vi "Query Bandwidth Part.vi"(6 "Carrier Component (1)":T2=1, 8 "error in (no error)":errorcluster, 9 "Bandwidth Part (BWP0)":T1 items=["BWP0"], 10 "Instance (1)":T3=1, 11 "VISA resource name":refnum<visa-resource-name>) -> (0 "error out":errorcluster, 1 "Cyclic Prefix":i32(ring) items=["Normal"], 2 "No Of RBs":i32=66, 3 "VISA resource name out":refnum<visa-resource-name>, 4 "Start RB":i32, 5 "Subcarrier Spacing":i32(ring)=1 items=["60 kHz", "120 kHz"])   [LabVIEW 2015, in "Rohde&Schwarz CMXP NR FR2 Measurement.lvlib"]
doc: "Queries basic properties of the <BWP> on carrier <CC>.\n\nAttribute:\n-\n\nRemote-control command:\nCONFigure:NRMMw:MEAS<i>[:CC<no>]:BWPart? <BWP>"
uses:
  <instrlib>/Rohde&Schwarz CMXP NR FR2 Measurement/Rohde&Schwarz CMXP NR FR2 Measurement.lvlib
  <instrlib>/Rohde&Schwarz CMXP NR FR2 Measurement/Private/_Instance.ctl
  <instrlib>/Rohde&Schwarz CMXP NR FR2 Measurement/Private/_Carrier Component.ctl
  <instrlib>/Rohde&Schwarz CMXP NR FR2 Measurement/Private/_Bandwidth Part.ctl
  <instrlib>/Rohde&Schwarz CMXP NR FR2 Measurement/Private/rsidr_core.llb/rsidr_core.lvlib
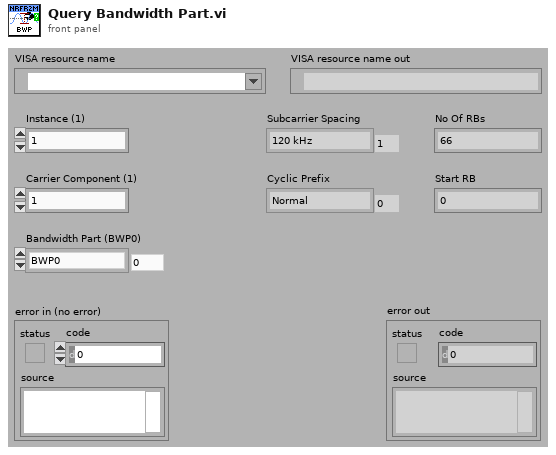
[diagram p1: front panel]
types:
  T1 = typedef "Rohde&Schwarz CMXP NR FR2 Measurement.lvlib/_Bandwidth Part.ctl" = i32
  T2 = typedef "Rohde&Schwarz CMXP NR FR2 Measurement.lvlib/_Carrier Component.ctl" = i32
  T3 = typedef "Rohde&Schwarz CMXP NR FR2 Measurement.lvlib/_Instance.ctl" = i32
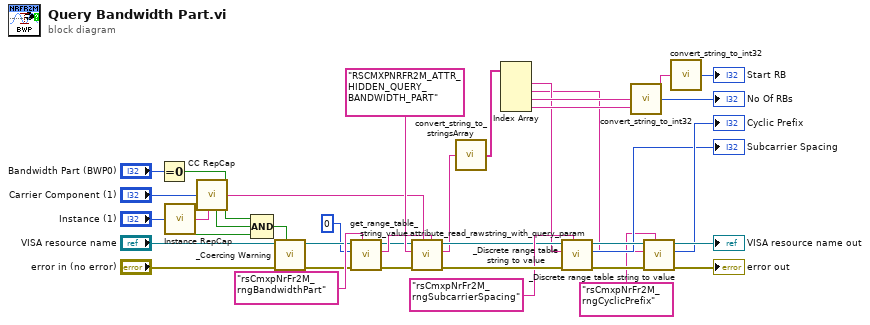
[diagram p0: block diagram]
diagram:
  n1 = Equal To 0?(x="Bandwidth Part (BWP0)") -> (x = 0?=w8:bool)
  n2 = call <instrlib>:"Instance RepCap.vi"("Instance In"="Instance (1)") -> ("In Range?"=w33:bool, "RepCap Identifier Out"=w6:string)  [unwired: 1 in]
  n3 = call <instrlib>:"CC RepCap.vi"("CC In"="Carrier Component (1)", "RepCap String In (\"\")"=w6) -> ("In Range?"=w32:bool, "RepCap Identifier Out"=w28:string)
  n4 = Compound Arithmetic op=AND(w8, w32, w33) -> (w35:bool)
  n5 = call <instrlib>:"_Coercing Warning.vi"("In Range?"=w35, "error in (no error)"="error in (no error)", "VISA resource name"="VISA resource name") -> ("error out"=w14:errorcluster, "VISA resource name out"=w13:refnum<visa-resource-name>)  [unwired: 7 in]
  n6 = call <instrlib>:"get_range_table_string_value.vi"("Range Table ID in"="rsCmxpNrFr2M_rngBandwidthPart", "error in"=w14, "I32 input"=0, "VISA resource name"=w13) -> ("error out"=w25:errorcluster, "String Value out"=w27:string, "VISA resource name out"=w26:refnum<visa-resource-name>)  [unwired: 5 in]
  n7 = call <instrlib>:"attribute_read_rawstring_with_query_param.vi"("Query Parameter (None)"=w27, "Repeated Capability"=w28, "error in"=w25, "Attribute ID"="RSCMXPNRFR2M_ATTR_HIDDEN_QUERY_BANDWIDTH_PART", "VISA resource name"=w26) -> ("error out"=w24:errorcluster, "Raw String out"=w12:string, "VISA resource name out"=w19:refnum<visa-resource-name>)  [unwired: 4 in]
  n8 = call <instrlib>:"convert_string_to_stringsArray.vi"("String in"=w12) -> ("string array out"=w11:string[])  [unwired: 3 in, 1 out]
  n9 = Index Array(array=w11) -> (element #1=w3:string, element #2=w2:string, element #3=w17:string, element #4=w4:string)  [unwired: 4 in]
  n10 = call <instrlib>:"_Discrete range table string to value.vi"("Discrete Range Table Identifier"="rsCmxpNrFr2M_rngSubcarrierSpacing", "error in (no error)"=w24, "String Value In"=w3, "VISA resource name"=w19) -> ("error out"=w21:errorcluster, "Enum Value"=→"Subcarrier Spacing":i32, "VISA resource name out"=w22:refnum<visa-resource-name>)  [unwired: 5 in]
  n11 = call <instrlib>:"convert_string_to_int32.vi"("String in"=w17) -> ("int32 value out"=→"No Of RBs":i32)  [unwired: 4 in]
  n12 = call <instrlib>:"_Discrete range table string to value.vi"("Discrete Range Table Identifier"="rsCmxpNrFr2M_rngCyclicPrefix", "error in (no error)"=w21, "String Value In"=w2, "VISA resource name"=w22) -> ("error out"=→"error out":errorcluster, "Enum Value"=→"Cyclic Prefix":i32, "VISA resource name out"=→"VISA resource name out":refnum<visa-resource-name>)  [unwired: 5 in]
  n13 = call <instrlib>:"convert_string_to_int32.vi"("String in"=w4) -> ("int32 value out"=→"Start RB":i32)  [unwired: 4 in]
